vi "Wf binary to float.vi"(2 "Input string":string) -> (16 "Data out":sgl[](array[numeric]))   [LabVIEW 2021, in "RedPitaya.lvlib"]
uses:
  RedPitaya.lvlib
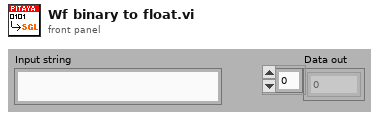
[diagram p1: front panel]
types:
  T1 = enum16{"big-endian, network order", "native, host order", "little-endian"}
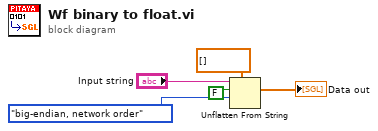
[diagram p0: block diagram]
diagram:
  n1 = Unflatten From String(type=sgl[] [] ("Si"), binary string="Input string", data includes array or string size? (T)=FALSE, byte order (0:big-endian, network order)=T1."big-endian, network order") -> (value=→"Data out":sgl[])  [unwired: 1 in, 2 out]
